vi "Create DVR.vi"(11 "error in (no error)":errorcluster) -> (4 "DVR Out":refnum<data-value>, 15 "error out":errorcluster)   [LabVIEW 2020, in "Communication.lvclass"]
doc: "Create Notifier object DVR."
uses:
  Classes/Communication/Communication.lvclass
panel:
  in  "DVR In":refnum<data-value>
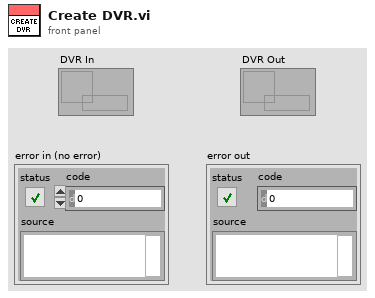
[diagram p1: front panel]
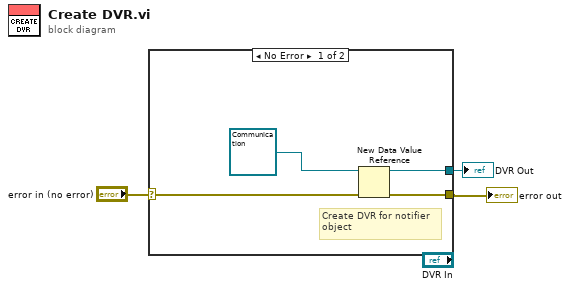
[diagram p0: block diagram]
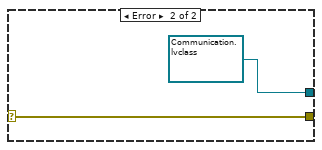
[diagram p2: hidden frame]
diagram:
  n1 = case shown="No Error" "error in (no error)" {
    selector: "error in (no error)" -> [w7 w9]
    tunnel: [w6 w9] -> w2
    tunnel: [w4 refnum<data-value> refnum ("data value reference")] -> w1
    frame No Error {
      # "Create DVR for notifier\nobject"
      n2 = New Data Value Reference(data value=refnum<class "Communication.lvclass"> refnum ("Communication.lvclass"), error in=w7) -> (data value reference=w4:refnum<data-value>, error out=w6:errorcluster)
    }
    frame Error {
    }
  }
  "error out" <- w2
  "DVR Out" <- w1
